vi "4 Axis - Get Axis Position.vi"(4 "error in (no error)":errorcluster, 7 "Controller Reference In":refnum<k7>) -> (0 "error out":errorcluster, 1 "Axis Positions":sgl[](array[numeric]), 3 "Controller Reference Out":refnum<k7>)   [LabVIEW 2015]
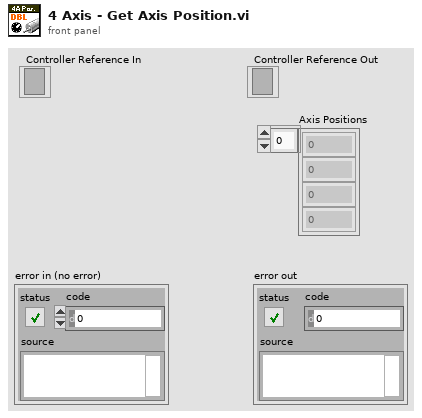
[diagram p1: front panel]
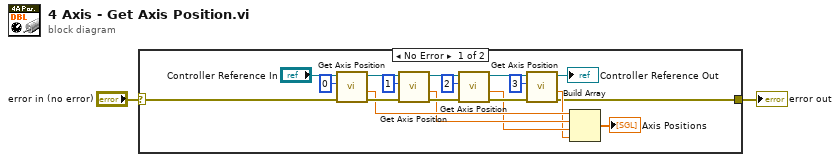
[diagram p0: block diagram]
diagram:
  n1 = case shown="No Error" "error in (no error)" {
    selector: "error in (no error)" -> [w3 w22]
    tunnel: [w5 w22] -> w2
    frame No Error {
      n2 = call "Get Axis Position.vi"("error in (no error)"=w3, "Axis In"=i16 0, "Controller Reference In"="Controller Reference In") -> ("error out"=w18:errorcluster, "Position Out"=w10:sgl, "Controller Reference Out"=w21:refnum<k7>)  [unwired: 1 in, 1 out]
      n3 = call "Get Axis Position.vi"("error in (no error)"=w18, "Axis In"=i16 1, "Controller Reference In"=w21) -> ("error out"=w17:errorcluster, "Position Out"=w9:sgl, "Controller Reference Out"=w20:refnum<k7>)  [unwired: 1 in, 1 out]
      n4 = call "Get Axis Position.vi"("error in (no error)"=w17, "Axis In"=i16 2, "Controller Reference In"=w20) -> ("error out"=w16:errorcluster, "Position Out"=w8:sgl, "Controller Reference Out"=w19:refnum<k7>)  [unwired: 1 in, 1 out]
      n5 = call "Get Axis Position.vi"("error in (no error)"=w16, "Axis In"=i16 3, "Controller Reference In"=w19) -> ("error out"=w5:errorcluster, "Position Out"=w7:sgl, "Controller Reference Out"=→"Controller Reference Out":refnum<k7>)  [unwired: 1 in, 1 out]
      n6 = Build Array(w10, w9, w8, w7) -> (→"Axis Positions":sgl[])
    }
    frame Error {
    }
  }
  "error out" <- w2
